vi "Timer.vi"(7 "ms":u32, 8 "Load (F)":bool, 9 "Reset (F)":bool, 10 "Start (T)":bool=TRUE) -> (2 "t ms":u32, 3 "End":bool)   [LabVIEW 2019, in "Timers.lvlib"]
uses:
  Timers.lvlib
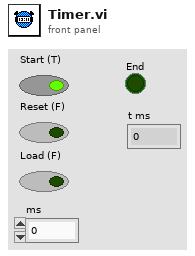
[diagram p1: front panel]
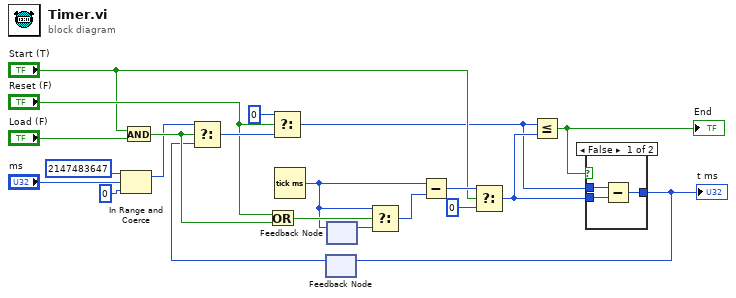
[diagram p0: block diagram]
diagram:
  n1 = In Range and Coerce(upper limit=u32 2147483647, x="ms", lower limit=u32 0) -> (coerced(x)=w5:u32)  [unwired: 1 out]
  n2 = And(x="Start (T)", y="Load (F)") -> (x .and. y?=w16:bool)
  n3 = Or(x="Reset (F)", y=w16) -> (x .or. y?=w21:bool)
  n4 = Tick Count (ms)() -> (millisecond timer value=w4:u32)
  n5 = feedback #1() -> (w1:u32)  [unwired: 1 in]
  n6 = Select(t=w5, s=w16, f=w1) -> (s? t:f=w19:u32)
  n7 = Select(t=u32 0, s="Reset (F)", f=w19) -> (s? t:f=w10:u32)
  n8 = feedback #2() -> (w3:u32)  [unwired: 1 in]
  n9 = feedback-in #2(w4) -> ()
  n10 = Select(t=w4, s=w21, f=w3) -> (s? t:f=w9:u32)
  n11 = Subtract(x=w4, y=w9) -> (x-y=w14:u32)
  n12 = Select(t=w14, s="Start (T)", f=u32 0) -> (s? t:f=w11:u32)
  n13 = Less Or Equal?(x=w10, y=w11) -> (x <= y?=w15:bool)
  "End" <- w15
  n14 = case shown="False" w15 {
    tunnel: w11 -> [w23 _]
    tunnel: [w24 _] -> w2
    tunnel: w10 -> [w22 _]
    frame False {
      n15 = Subtract(x=w22, y=w23) -> (x-y=w24:u32)
    }
    frame True {
    }
  }
  "t ms" <- w2
  n16 = feedback-in #1(w2) -> ()
